vi "ProdaNG.Convert.String-I32.vi"(11 "unsigned byte string":string) -> (3 "32bit integer":i32)   [LabVIEW 2016]
panel:
  # "s"
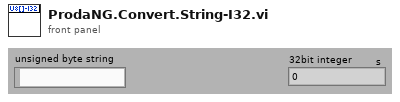
[diagram p1: front panel]
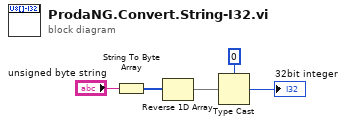
[diagram p0: block diagram]
diagram:
  n1 = String To Byte Array(string="unsigned byte string") -> (unsigned byte array=w4:u8[])
  n2 = Reverse 1D Array(array=w4) -> (reversed array=w3:u8[])
  n3 = Type Cast(type=0 ("32bit integer"), x=w3) -> (*(type *) &x=→"32bit integer":i32)
